vi "Get Moddule ID to Stop Instance.vi"(8 "error in":errorcluster, 10 "Remote Port":u16, 11 "Remote IP":string) -> (0 "error out":errorcluster, 2 "index of element":i32, 3 "Module ID to be deleted":i32)   [LabVIEW 2021, in "RT Interpreter Manager.lvlib"]
uses:
  RT Interpreter Manager.lvlib
  RT Interpreter.lvlib
  Clone Registration/Clone Registration.lvlib
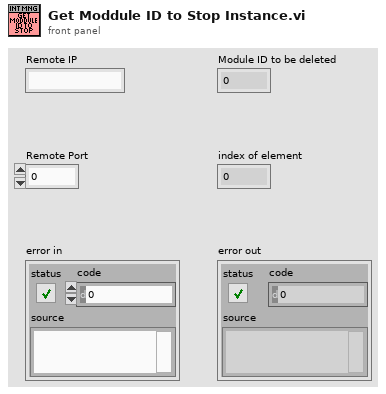
[diagram p1: front panel]
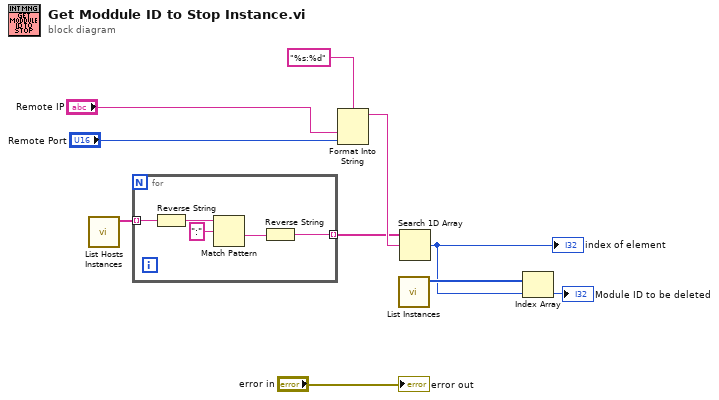
[diagram p0: block diagram]
diagram:
  n1 = call "List Hosts Instances.vi"() -> ("List of IP:Port:Master/Slave"=w10:string[])  [unwired: 10 in, 1 out]
  n2 = for {
    tunnel: w10 -> [w15] mode=indexing
    tunnel: [w11] -> w5 mode=indexing
    n3 = Reverse String(1:w15) -> (0:w14:string)
    n4 = Match Pattern(string=w14, regular expression=":") -> (after substring=w12:string)  [unwired: 1 in, 3 out]
    n5 = Reverse String(1:w12) -> (0:w11:string)
  }
  n6 = Format Into String(format string="%s:%d", "Remote IP", "Remote Port") -> (resulting string=w6:string)  [unwired: 2 in, 1 out]
  n7 = call "List Instances.vi"() -> ("Module IDs"=w4:i32[])  [unwired: 7 in, 4 out]
  n8 = Search 1D Array(1D array=w5, element=w6) -> (index of element=w3:i32)  [unwired: 1 in]
  "index of element" <- w3
  n9 = Index Array(array=w4, index=w3) -> (element=→"Module ID to be deleted":i32)
  "error out" <- "error in"
